vi "Enum from Value.vi"(10 "Value":i32) -> (2 "Enumeration":T1)   [LabVIEW 2020, in "EventLevel.lvlib"]
uses:
  EventLevel.lvlib
  Enumeration.ctl
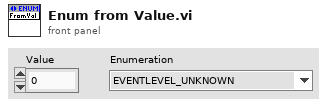
[diagram p1: front panel]
types:
  T1 = typedef "EventLevel.lvlib/Enumeration.ctl" = enum16{"EVENTLEVEL_UNKNOWN", "EVENTLEVEL_DEBUG", "EVENTLEVEL_INFO", "EVENTLEVEL_WARNING", "EVENTLEVEL_ERROR"}
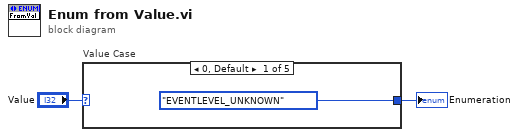
[diagram p0: block diagram]
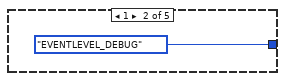
[diagram p2: hidden frame]
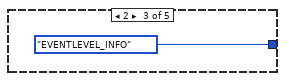
[diagram p3: hidden frame]
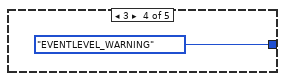
[diagram p4: hidden frame]
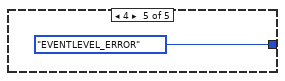
[diagram p5: hidden frame]
diagram:
  n1 = case "Value Case" shown="0, Default" "Value" {
    tunnel: [Enumeration."EVENTLEVEL_UNKNOWN" ("Enumeration") Enumeration."EVENTLEVEL_DEBUG" ("Enumeration") Enumeration."EVENTLEVEL_INFO" ("Enumeration") Enumeration."EVENTLEVEL_WARNING" ("Enumeration") Enumeration."EVENTLEVEL_ERROR" ("Enumeration")] -> w1
    frame 0, Default {
    }
    frame 1 {
    }
    frame 2 {
    }
    frame 3 {
    }
    frame 4 {
    }
  }
  "Enumeration" <- w1
